vi "SNR.vi"(11 "Array":dbl[](array[numeric])) -> (1 "方差":dbl, 2 "Amplitude":dbl, 3 "SNR":dbl)   [LabVIEW 2014]
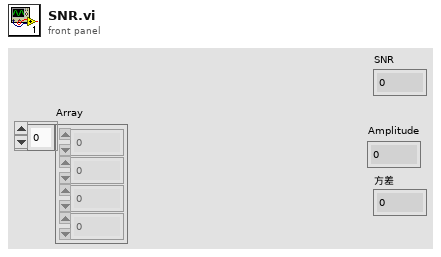
[diagram p1: front panel]
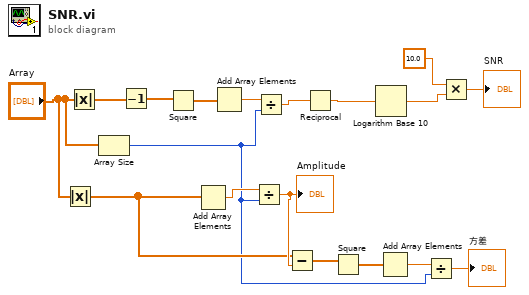
[diagram p0: block diagram]
diagram:
  n1 = Absolute Value(x="Array") -> (abs(x)=w6:dbl[])
  n2 = Absolute Value(x="Array") -> (abs(x)=w18:dbl[])
  n3 = Array Size(array="Array") -> (size(s)=w2:i32)
  n4 = Decrement(x=w18) -> (x-1=w17:dbl[])
  n5 = Square(x=w17) -> (x^2=w16:dbl[])
  n6 = Add Array Elements(numeric array=w6) -> (sum=w9:dbl)
  n7 = Add Array Elements(numeric array=w16) -> (sum=w11:dbl)
  n8 = Divide(x=w9, y=w2) -> (x/y=w8:dbl)
  "Amplitude" <- w8
  n9 = Divide(x=w11, y=w2) -> (x/y=w10:dbl)
  n10 = Subtract(x=w6, y=w8) -> (x-y=w5:dbl[])
  n11 = Reciprocal(x=w10) -> (1/x=w15:dbl)
  n12 = Square(x=w5) -> (x^2=w4:dbl[])
  n13 = Logarithm Base 10(1:w15) -> (0:w14:dbl)
  n14 = Add Array Elements(numeric array=w4) -> (sum=w3:dbl)
  n15 = Divide(x=w3, y=w2) -> (x/y=→"方差":dbl)
  n16 = Multiply(x=10.0, y=w14) -> (x*y=→"SNR":dbl)
